vi "Latch.vi"(8 "Reset":bool, 11 "Input":dbl format="%#_13g") -> (3 "Output":dbl format="%#_13g")   [LabVIEW 2014]
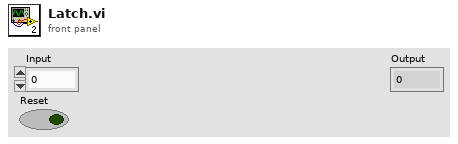
[diagram p1: front panel]
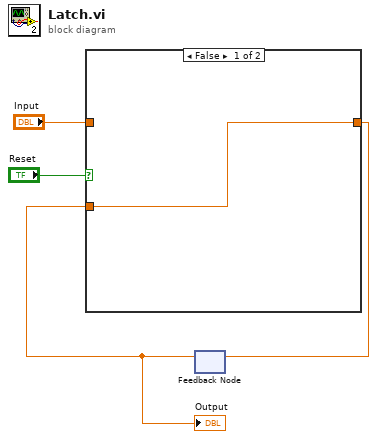
[diagram p0: block diagram]
diagram:
  n1 = feedback #1() -> (w2:dbl)  [unwired: 1 in]
  "Output" <- w2
  n2 = case shown="False" "Reset" {
    tunnel: "Input" -> [_ w6]
    tunnel: w2 -> [w5 _]
    tunnel: [w5 w6] -> w1
    frame False {
    }
    frame True {
    }
  }
  n3 = feedback-in #1(w1) -> ()
